vi "Update Front Panel.vi"(8 "error in (no error)":errorcluster, 11 "MediatorBusMonitor In":refnum<class "MediatorBusMonitor.lvclass">) -> (0 "error out":errorcluster, 3 "MediatorBusMonitor Out":refnum<class "MediatorBusMonitor.lvclass">)   [LabVIEW 2015, in "Mediator.lvlib" / "MediatorBusMonitor.lvclass"]
uses:
  MediatorBusMonitor/MediatorBusMonitor.lvclass
  MediatorBusMonitor/MediatorBusMonitor.lvclass/MediatorBusMonitor.ctl
  Components/VariantExtensions/Scalar Data to String.vi
  <vilib>/Utility/Data Type/Get Type Information.vi
  Components/CurrentValueTable/CurrentValueTable.lvclass
  Components/VariantExtensions/VariantExtensions.lvlib
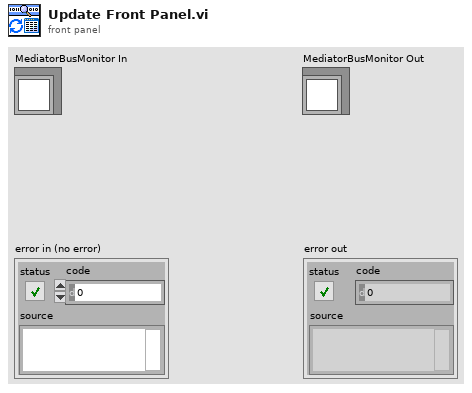
[diagram p1: front panel]
types:
  T1 = typedef "CurrentValueTable.lvlib/CurrentValueTable.lvclass/CurrentValueTable Reference.ctl" = refnum<data-value>
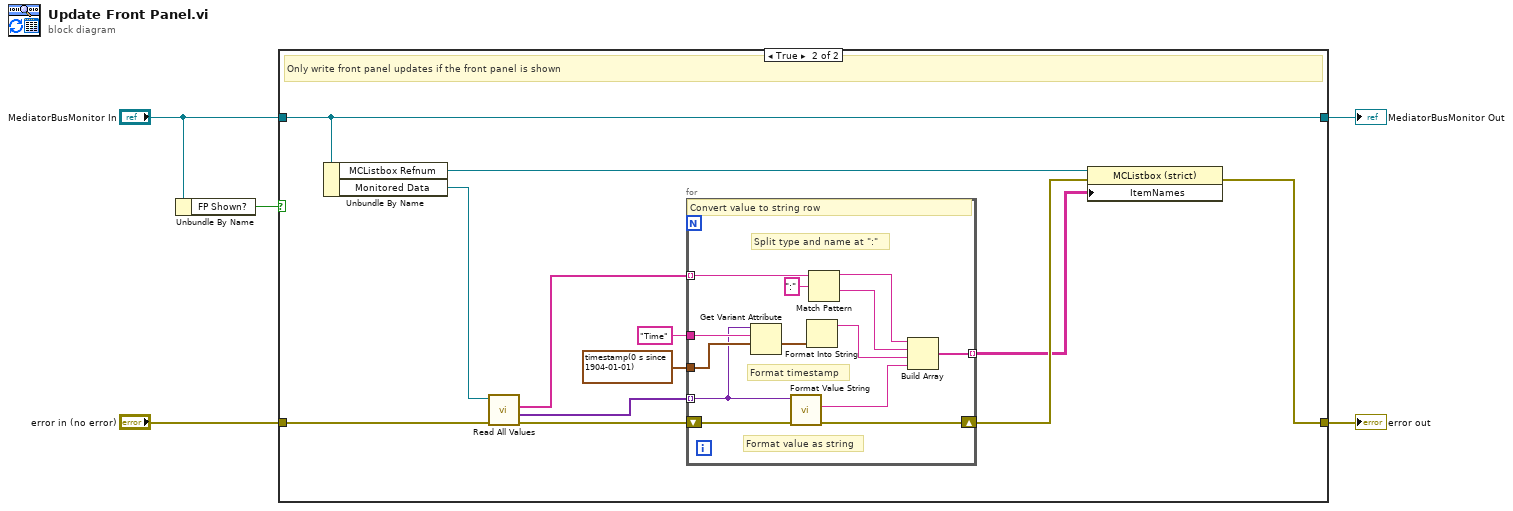
[diagram p0: block diagram]
diagram:
  n1 = Unbundle By Name("MediatorBusMonitor In") -> ("FP Shown?"=w3:bool)
  n2 = case shown="True" w3 {
    tunnel: "MediatorBusMonitor In" -> [w7 w12]
    tunnel: [w7 w12] -> w5
    tunnel: "error in (no error)" -> [w6 w16]
    tunnel: [w6 w13] -> w1
    frame False {
    }
    frame True {
      # "Only write front panel updates if the front panel is shown"
      n3 = Unbundle By Name(w12) -> ("MCListbox Refnum"=w19:refnum<vi>, "Monitored Data"=w18:T1)
      n4 = call "Read All Values.vi"("error in (no error)"=w16, "Current Value Table"=w18) -> ("error out"=w15:errorcluster, "Values"=w17:variant[], "Names"=w11:string[])  [unwired: 6 in, 1 out]
      n5 = for {
        tunnel: w17 -> [w20] mode=indexing
        shift-right: [w22] -> w14
        shift-left: w15 -> [w23]
        tunnel: w11 -> [w28] mode=indexing
        tunnel: timestamp(0 s since 1904-01-01) -> [w30]
        tunnel: [w24] -> w9 mode=indexing
        tunnel: "Time" ("name") -> [w21]
        # "Format timestamp"
        # "Format value as string"
        # "Split type and name at \":\""
        # "Convert value to string row"
        n6 = Get Variant Attribute(Variant=w20, name=w21, default value (empty Variant)=w30) -> (value=w29:timestamp)  [unwired: 1 in, 3 out]
        n7 = call "Format Value String.vi"("error in (no error)"=w23, "Data"=w20) -> ("error out"=w22:errorcluster, "Value as String"=w31:string)  [unwired: 8 in]
        n8 = Format Into String(w29) -> (resulting string=w32:string)  [unwired: 3 in, 1 out]
        n9 = Match Pattern(string=w28, regular expression=":" ("search string/char (-)")) -> (before substring=w26:string, after substring=w25:string)  [unwired: 1 in, 2 out]
        n10 = Build Array(w26, w25, w32, w31) -> (w24:string[])
      }
      n11 = property class="MCListbox (strict)"(reference=w19, error in=w14, "ItemNames"=w9) -> (error out=w13:errorcluster)  [unwired: 1 out]
    }
  }
  "MediatorBusMonitor Out" <- w5
  "error out" <- w1
